vi "WAM_BarCode_Prompt.vi"(0 "Enable":bool=TRUE, 11 "error in (no error)":errorcluster, 12 "Rev_suffix":string) -> (1 "Bar Code":string, 2 "BarCodeInfo":string, 3 "BC_MSN":string, 4 "cancelled?(t)":bool, 6 "LotID":string, 8 "rev_c?(t)":bool, 13 "BC_ESN":string, 14 "Revision":string, 15 "error out":errorcluster)   [LabVIEW 2018]
panel:
  out "Success?(t)":bool
  out "Rage Bar Code?(t)":bool
  out "Leidos Bar Code?(t)":bool
  out "Company":string
  out "Rage PN":string
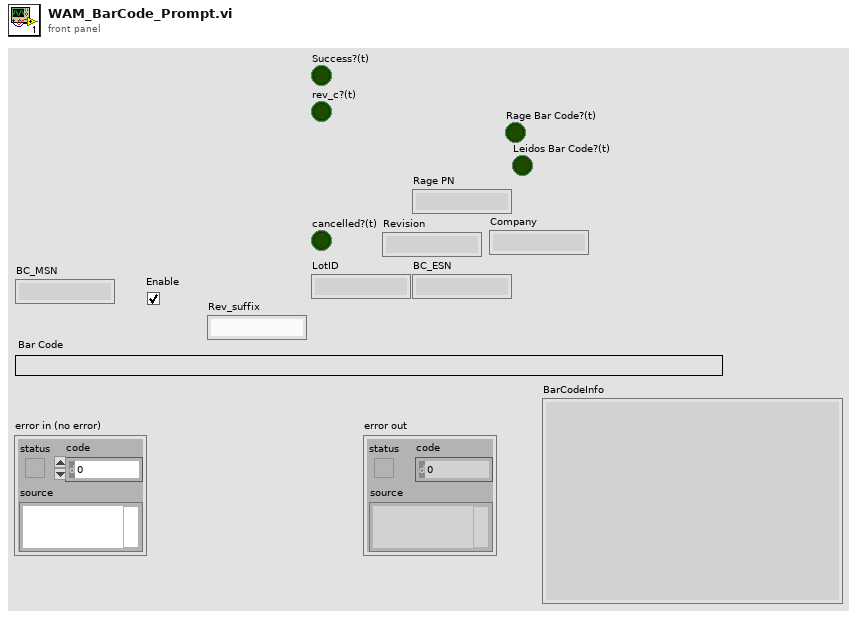
[diagram p1: front panel]
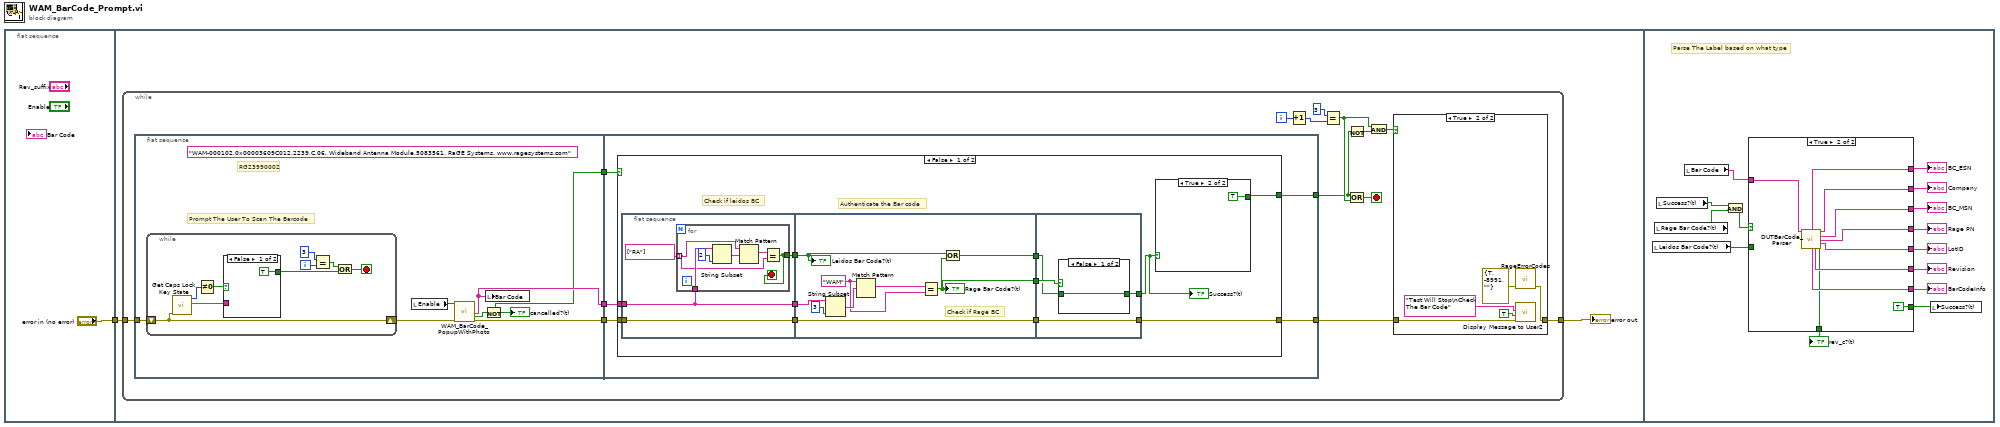
[diagram p0: block diagram]
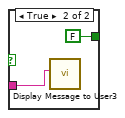
[diagram p3: hidden frame]
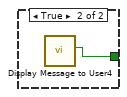
[diagram p4: hidden frame]
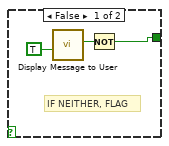
[diagram p5: hidden frame]
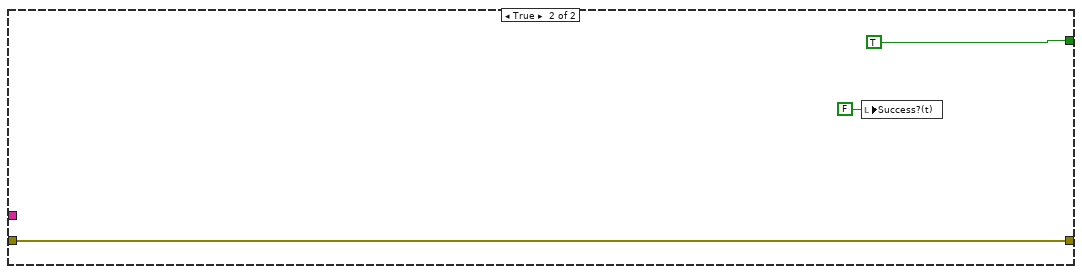
[diagram p6: hidden frame]
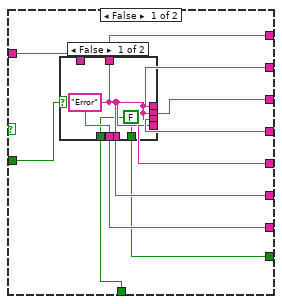
[diagram p7: hidden frame]
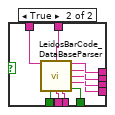
[diagram p8: hidden frame]
diagram:
  n1 = flat-sequence {
    tunnel: ["error in (no error)"] -> w1
    tunnel: w1 -> [w3]
    frame #0 {
    }
    frame #1 {
      n2 = while {
        tunnel: [w12] -> w4
        tunnel: w3 -> [w5]
        i -> [w17]
        stop <- w10 stop-if-true
        n3 = flat-sequence {
          tunnel: [w26] -> w18
          tunnel: [w25] -> w15
          tunnel: [w29] -> w14
          tunnel: w5 -> [w28]
          tunnel: [w48] -> w7
          tunnel: w18 -> [w46]
          tunnel: w15 -> [w47]
          tunnel: w14 -> [w45]
          tunnel: [w44] -> w13
          frame #0 {
            (unwired) "WAM-000102,0x00003609C012,2239,C.06, Wideband Antenna Module,5083561, RaGE Systems, www.ragesystems.com" ("Bar Code")
            # "RG23990002"
            # "Prompt The User To Scan The Barcode"
            n4 = while {
              shift-right: [w32] -> w30
              shift-left: w28 -> [w32]
              i -> [w35]
              stop <- w36 stop-if-true
              n5 = call "Get Caps Lock Key State.vi"("Error In"=w32) -> ("Caps Lock Key State (Text)"=w37:string, "Caps Lock Key State (Numeric)"=w40:i16)  [unwired: 8 in, 1 out]
              n6 = Not Equal To 0?(x=w40) -> (x != 0?=w39:bool)
              n7 = case shown="False" w39 {
                tunnel: [TRUE FALSE] -> w38
                tunnel: w37 -> [_ w43]
                frame False {
                }
                frame True {
                  n8 = call "Display Message to User3"("Message"=w43) -> ()  [unwired: 9 in, 2 out]
                }
              }
              n9 = Equal?(x=3, y=w35) -> (x = y?=w33:bool)
              n10 = Or(x=w33, y=w38) -> (x .or. y?=w36:bool)
            }
            n11 = local read "Enable"() -> (w27:bool)
            n12 = call "WAM_BarCode_PopupWithPhoto.vi"("Enable"=w27, "error in (no error)"=w30) -> ("Bar Code"=w26:string, "OK"=w31:bool, "error out"=w29:errorcluster)  [unwired: 14 in, 1 out]
            n13 = Not(x=w31) -> (.not. x?=w25:bool)
            "cancelled?(t)" <- w25
            n14 = local write "Bar Code"(w26) -> ()
          }
          frame #1 {
            n15 = case shown="False" w47 {
              tunnel: w46 -> [w58 _]
              tunnel: [w59 TRUE] -> w48
              tunnel: w45 -> [w55 w90]
              tunnel: [w53 w90] -> w44
              frame False {
                # "Check if leidos BC"
                # "Authenticate the Bar code"
                n16 = flat-sequence {
                  tunnel: w58 -> [w63]
                  tunnel: [w63] -> w57
                  tunnel: [w62] -> w56
                  tunnel: w55 -> [w61]
                  tunnel: [w61] -> w54
                  tunnel: w57 -> [w78]
                  tunnel: w56 -> [w73]
                  tunnel: w54 -> [w71]
                  tunnel: [w72] -> w52
                  tunnel: [w71] -> w51
                  tunnel: [w70] -> w50
                  tunnel: [w82] -> w53
                  tunnel: w52 -> [w79]
                  tunnel: w51 -> [w82]
                  tunnel: w50 -> [w81]
                  tunnel: [w80] -> w49
                  frame #0 {
                    n17 = for {
                      tunnel: w63 -> [w66]
                      tunnel: [w64] -> w62
                      tunnel: string[] ["RA"] ("string") -> [w65] mode=indexing
                      stop <- w64 stop-if-true
                      n18 = String Subset(string=w66, length (rest)=2 ("length (rest)")) -> (substring=w68:string)  [unwired: 1 in]
                      n19 = Match Pattern(string=w65, regular expression=w68) -> (match substring=w69:string)  [unwired: 1 in, 3 out]
                      n20 = Equal?(x=w69, y=w65) -> (x = y?=w64:bool)
                    }
                  }
                  frame #1 {
                    w74 = "WAM" ("string")
                    # "Check if Rage BC"
                    n21 = String Subset(string=w78, length (rest)=3 ("length (rest)")) -> (substring=w76:string)  [unwired: 1 in]
                    n22 = Match Pattern(string=w74, regular expression=w76) -> (match substring=w75:string)  [unwired: 1 in, 3 out]
                    n23 = Equal?(x=w75, y=w74) -> (x = y?=w70:bool)
                    "Rage Bar Code?(t)" <- w70
                    n24 = Or(x=w73, y=w70) -> (x .or. y?=w72:bool)
                    "Leidos Bar Code?(t)" <- w73
                  }
                  frame #2 {
                    n25 = case shown="False" w81 {
                      tunnel: [w83 w84] -> w80
                      tunnel: w79 -> [w83 _]
                      frame False {
                      }
                      frame True {
                        n26 = call "Display Message to User4"() -> ("OK"=w84:bool)  [unwired: 10 in, 1 out]
                      }
                    }
                  }
                }
                n27 = case shown="True" w49 {
                  tunnel: [w86 TRUE] -> w59
                  frame False {
                    # "IF NEITHER, FLAG"
                    n28 = call "Display Message to User"("Enable"=TRUE) -> ("OK"=w87:bool)  [unwired: 9 in, 1 out]
                    n29 = Not(x=w87) -> (.not. x?=w86:bool)
                  }
                  frame True {
                  }
                }
                "Success?(t)" <- w49
              }
              frame True {
                n30 = local write "Success?(t)"(FALSE ("Success?(t)")) -> ()
              }
            }
          }
        }
        n31 = Increment(x=w17) -> (x+1=w16:i32)
        n32 = Equal?(x=3, y=w16) -> (x = y?=w9:bool)
        n33 = Not(x=w7) -> (.not. x?=w6:bool)
        n34 = Or(x=w7, y=w9) -> (x .or. y?=w10:bool)
        n35 = And(x=w9, y=w6) -> (x .and. y?=w8:bool)
        n36 = case shown="True" w8 {
          tunnel: w13 -> [w19 w22]
          tunnel: [w19 w20] -> w12
          frame False {
          }
          frame True {
            n37 = call "RageErrorCodes.vi"("error in"=errorcluster {"status"=TRUE, "code"=-8991, "source"=""} ("error out")) -> ("error out"=w20:errorcluster)  [unwired: 8 in, 2 out]
            n38 = call "Display Message to User2"("error in (no error)"=w22, "Enable"=TRUE, "Message"="Test Will Stop\nCheck The Bar Code") -> ()  [unwired: 7 in, 2 out]
          }
        }
      }
      "error out" <- w4
    }
    frame #2 {
      # "Parse The Label based on what type"
      n39 = local read "Leidos Bar Code?(t)"() -> (w94:bool)
      n40 = local read "Rage Bar Code?(t)"() -> (w105:bool)
      n41 = local read "Success?(t)"() -> (w103:bool)
      n42 = local read "Bar Code"() -> (w95:string)
      n43 = And(x=w103, y=w105) -> (x .and. y?=w104:bool)
      n44 = case shown="True" w104 {
        tunnel: [w110 w138] -> w102
        tunnel: [w115 w137] -> w101
        tunnel: [w109 w136] -> w100
        tunnel: [w112 w135] -> w99
        tunnel: [w111 w134] -> w98
        tunnel: [w113 w133] -> w97
        tunnel: [w114 w132] -> w96
        tunnel: w95 -> [w116 w131]
        tunnel: w94 -> [w108 _]
        tunnel: [w107 TRUE ("Success?(t)")] -> w93
        tunnel: [w106 w129] -> w92
        frame False {
          n45 = case shown="False" w108 {
            tunnel: w116 -> [_ w128]
            tunnel: [w118 w127] -> w115
            tunnel: [w118 w126] -> w114
            tunnel: [w118 w125] -> w113
            tunnel: [w118 w124] -> w112
            tunnel: [w118 w123] -> w111
            tunnel: [w118 w122] -> w110
            tunnel: [w118 w121] -> w109
            tunnel: [w117 w120] -> w107
            tunnel: [w117 w119] -> w106
            frame False {
              w117 = FALSE ("Success?(t)")
              w118 = "Error" ("BarCodeInfo")
            }
            frame True {
              n46 = call "LeidosBarCode_DataBaseParser.vi"("BarCode_In"=w128) -> ("BC_ESN"=w121:string, "Company"=w127:string, "BC_MSN"=w126:string, "Rage PN"=w125:string, "LotID"=w124:string, "rev_c?(t)"=w119:bool, "BarCodeInfo"=w122:string, "Revision"=w123:string, "Success?(t)"=w120:bool)  [unwired: 4 in, 2 out]
            }
          }
        }
        frame True {
          n47 = call "DUTBarCode_Parser.vi"("DUT INFO"=w131) -> ("BC_ESN"=w136:string, "Company"=w137:string, "BC_MSN"=w132:string, "Rage PN"=w133:string, "LotID"=w135:string, "BarCodeInfo"=w138:string, "Revision"=w134:string, "rev_c?(t)"=w129:bool)  [unwired: 5 in, 2 out]
        }
      }
      "BC_MSN" <- w96
      "Rage PN" <- w97
      "Revision" <- w98
      "LotID" <- w99
      "BC_ESN" <- w100
      "Company" <- w101
      "BarCodeInfo" <- w102
      "rev_c?(t)" <- w92
      n48 = local write "Success?(t)"(w93) -> ()
    }
  }
